vi "Stop Core.vi"(10 "final error code":i32, 11 "WebSocket Server in":refnum<class "WebSocket Server.lvclass">) -> (3 "WebSocket Server out":refnum<class "WebSocket Server.lvclass">)   [LabVIEW 2016, in "WebSocket Actors.lvlib" / "WebSocket Server.lvclass"]
doc: "(<B>Filename</B>: Actor Framework.lvlib:Actor.lvclass:Stop Core.vi)\n\nDefines what the actor does before it stops. Use the <B>final error code</B> input to determine whether the actor shut down in response to an error.\n\nBy default, this method does nothing. A descendant class may override it to define behavior, such as shutting down any processes the actor initiated in its override of the Actor Core method."
uses:
  WebSocket Server.lvclass
  WebSocket Server.lvclass/WebSocket Server.ctl
  <vilib>/MGI/Monitored Actor/Monitored Actor/Monitored Actor/Monitored Actor.lvclass
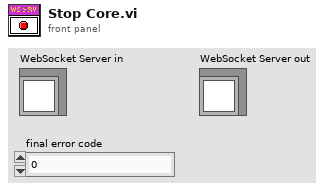
[diagram p1: front panel]
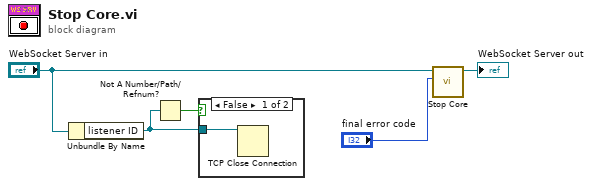
[diagram p0: block diagram]
diagram:
  n1 = Unbundle By Name("WebSocket Server in") -> ("listener ID"=w1:refnum<k5>)
  n2 = Not A Number/Path/Refnum?(number/path/refnum=w1) -> (NaN/Path/Refnum?=w2:bool)
  n3 = case shown="False" w2 {
    tunnel: w1 -> [w6 _]
    frame False {
      n4 = TCP Close Connection(connection ID=w6) -> ()  [unwired: 2 in, 2 out]
    }
    frame True {
    }
  }
  n5 = call-parent "Stop Core.vi"("final error code"="final error code", "Monitored Actor in"="WebSocket Server in") -> ("Monitored Actor out"=→"WebSocket Server out":refnum<class "WebSocket Server.lvclass">)  [unwired: 9 in]
